vi "SetSlitwidth.vi"(8 "error in (no error)":errorcluster, 9 "Slitwidth":u16, 10 "Slit":T1, 11 "HRS_Spectrometer in":refnum<class "HRS_Spectrometer.lvclass">) -> (0 "error out":errorcluster, 3 "HRS_Spectrometer out":refnum<class "HRS_Spectrometer.lvclass">)   [LabVIEW 2023, in "HRS_Spectrometer.lvlib" / "HRS_Spectrometer.lvclass"]
uses:
  HRS_Spectrometer.lvclass
  typedefs/SpectrSlitControl.ctl
  HRS_Spectrometer.lvclass/HRS_Spectrometer.ctl
  Interfaces/AbstractInstrumentClasses/Spectrometers_LV/SpectrometerComm Messages/SlitMoved Msg/SlitMoved Msg.lvclass/SlitMoved Msg.ctl
  <vilib>/ActorFramework/Message Enqueuer/Message Enqueuer.lvclass/Message Enqueuer.ctl
  <vilib>/ActorFramework/Message Enqueuer/Enqueue.vi
  Interfaces/AbstractInstrumentClasses/Spectrometers_LV/SpectrometerComm Messages/SlitMoved Msg/SlitMoved Msg.lvclass
  C:/Program Files/National Instruments/LabVIEW 2023/vi.lib/ActorFramework/Message/Message.lvclass
  <vilib>/ActorFramework/Message Priority Queue/Priority Enqueue.vi
  <vilib>/ActorFramework/Actor/Actor.lvclass
  C:/Program Files/National Instruments/LabVIEW 2023/vi.lib/ActorFramework/Actor/Actor.lvclass
  C:/Users/DELL/Documents/LVDAQ/ConcreteClasses/ConcreteInstrumentClasses/SpectrometerClasses/Spectrometer_HRS_LV/HRS_Spectrometer/HRS_Spectrometer/HRS_Spectrometer.lvclass
  C:/Users/DELL/Documents/LVDAQ/Interfaces/InitDeinitInterface/InitDeinit/InitDeinit.lvclass
  C:/Users/DELL/Documents/LVDAQ/Interfaces/AbstractInstrumentClasses/Spectrometers_LV/SpectrometerInterface/Spectrometer.lvclass
  typedefs/typedefs.lvlib
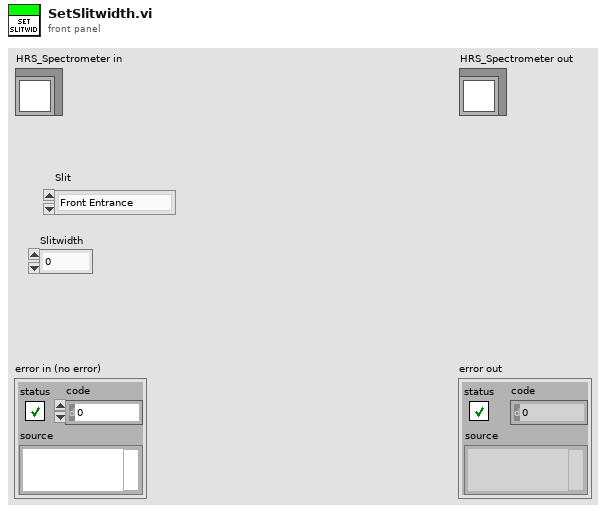
[diagram p1: front panel]
types:
  T1 = typedef "typedefs.lvlib/SpectrSlitControl.ctl" = enum16{"Front Entrance", "Side Entrance", "Front Exit", "Side Exit"}
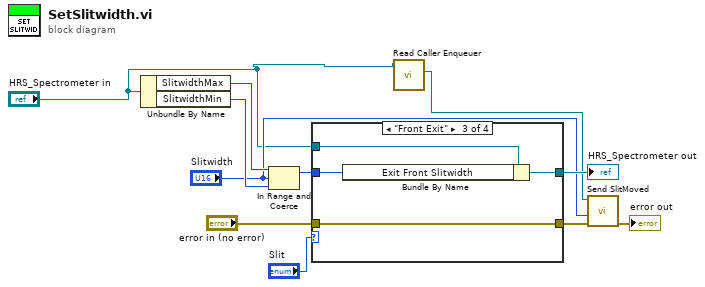
[diagram p0: block diagram]
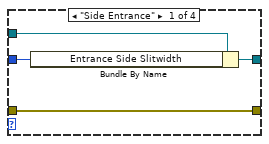
[diagram p2: hidden frame]
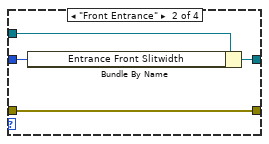
[diagram p3: hidden frame]
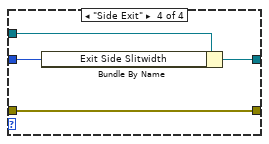
[diagram p4: hidden frame]
diagram:
  n1 = Unbundle By Name("HRS_Spectrometer in") -> ("SlitwidthMax"=w11:u16, "SlitwidthMin"=w10:u16)
  n2 = In Range and Coerce(upper limit=w11, x="Slitwidth", lower limit=w10) -> (coerced(x)=w7:u16)  [unwired: 1 out]
  n3 = case shown="\"Front Exit\"" "Slit" {
    tunnel: "HRS_Spectrometer in" -> [w15 w19 w23 w27]
    tunnel: [w14 w18 w22 w26] -> w9
    tunnel: w7 -> [w13 w17 w21 w25]
    tunnel: "error in (no error)" -> [w12 w16 w20 w24]
    tunnel: [w12 w16 w20 w24] -> w4
    frame "Side Entrance" {
      n4 = Bundle By Name(cluster=w15, "Entrance Side Slitwidth"=w13) -> (w14:refnum<class "HRS_Spectrometer.lvclass">)
    }
    frame "Front Entrance" {
      n5 = Bundle By Name(cluster=w19, "Entrance Front Slitwidth"=w17) -> (w18:refnum<class "HRS_Spectrometer.lvclass">)
    }
    frame "Front Exit" {
      n6 = Bundle By Name(cluster=w23, "Exit Front Slitwidth"=w21) -> (w22:refnum<class "HRS_Spectrometer.lvclass">)
    }
    frame "Side Exit" {
      n7 = Bundle By Name(cluster=w27, "Exit Side Slitwidth"=w25) -> (w26:refnum<class "HRS_Spectrometer.lvclass">)
    }
  }
  "HRS_Spectrometer out" <- w9
  n8 = call <vilib>:"Read Caller Enqueuer.vi"("Actor"="HRS_Spectrometer in") -> ("Caller Enqueuer"=w2:refnum<class "Message Enqueuer.lvclass">)  [unwired: 10 in]
  n9 = call "Send SlitMoved.vi"("error in (no error)"=w4, "Slitwidth"="Slitwidth", "Message Enqueuer"=w2) -> ("error out"=→"error out":errorcluster)  [unwired: 7 in, 1 out]
